vi "GhostShoot.vi"(10 "Robot":T1, 11 "Buttons":bool[](array[boolean])) -> ()   [LabVIEW 2015]
uses:
  Robot Type Def.ctl
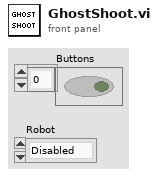
[diagram p1: front panel]
types:
  T1 = typedef "Robot Type Def.ctl" = enum32{"Disabled", "Ghost", "Casper", "Lofty", "Board", "RaceRobot", "Casper 2.0", "Excalibot 2.0"}
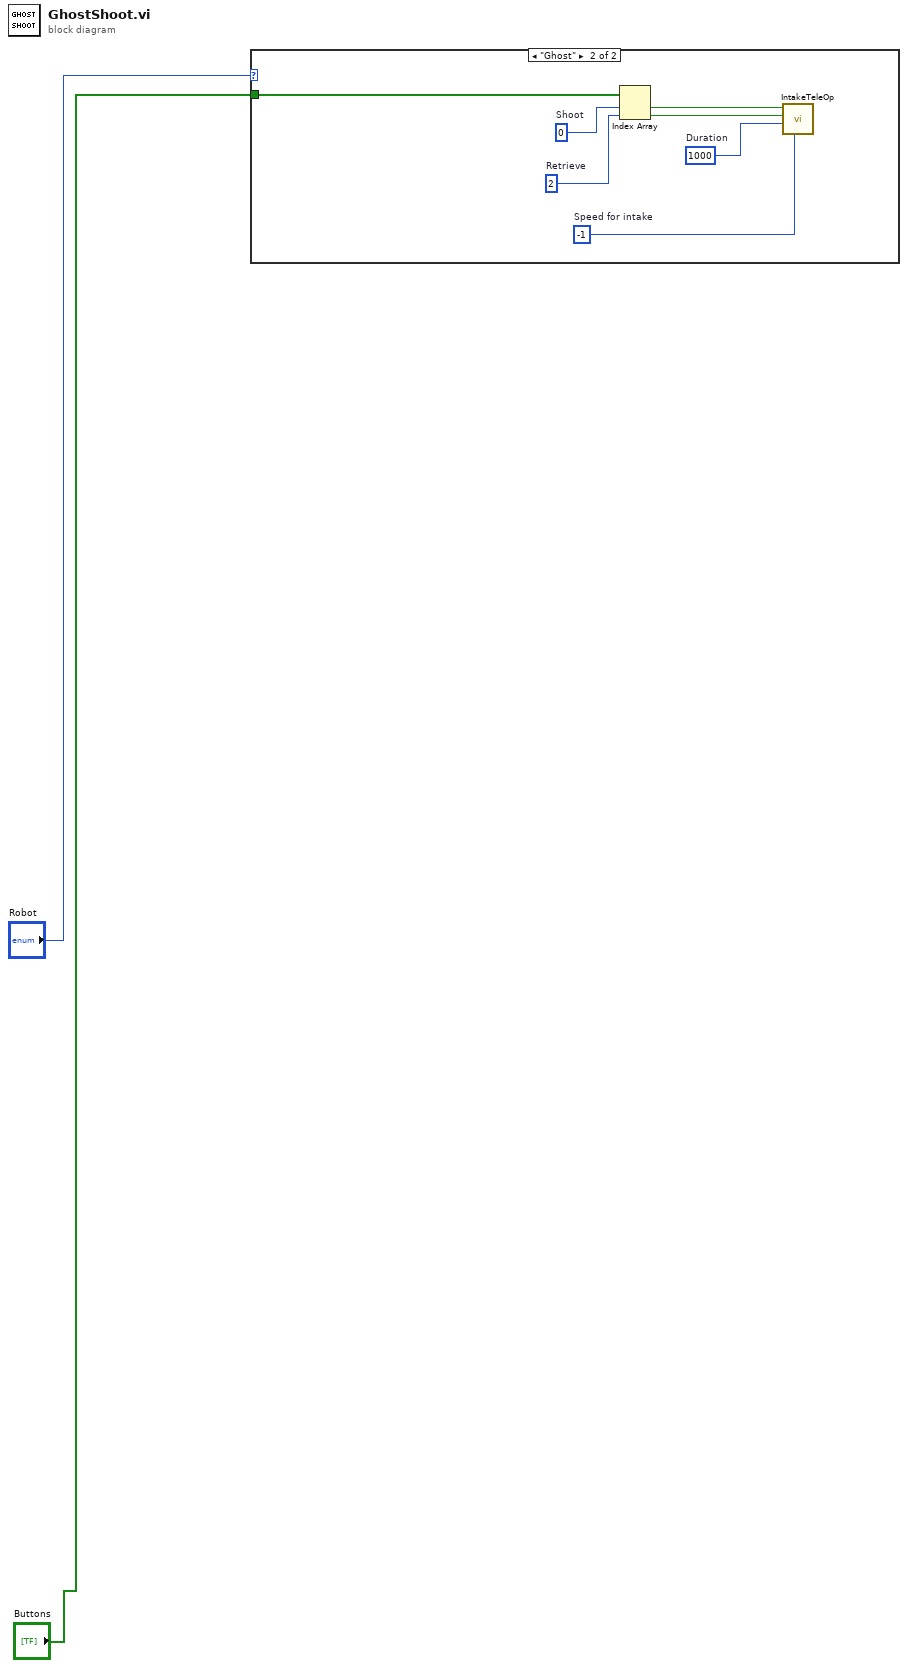
[diagram p0: block diagram]
diagram:
  n1 = case shown="\"Ghost\"" "Robot" {
    tunnel: "Buttons" -> [_ w4]
    frame "Disabled", Default {
    }
    frame "Ghost" {
      w7 = 1000  # Duration
      w6 = 2  # Retrieve
      w5 = 0  # Shoot
      w3 = -1  # Speed for intake
      n2 = Index Array(array=w4, index #1=w5, index #2=w6) -> (element #1=w8:bool, element #2=w9:bool)
      n3 = call "IntakeTeleOp.vi"("Speed for intake"=w3, "Duration"=w7, "Retrieve"=w9, "Shoot"=w8) -> ()  [unwired: 8 in]
    }
  }
